vi "Cleanup.vi"(8 "error in (no error)":errorcluster, 11 "SQLite in":refnum<class "SQLite.lvclass">) -> (0 "error out":errorcluster)   [LabVIEW 2020, in "Summer of LabVIEW.lvlib" / "SQLite.lvclass"]
uses:
  SQLite.lvclass
  SQLite.lvclass/SQLite.ctl
  <vilib>/drjdpowell/SQLite Library/SQL Connection/Connection.lvclass
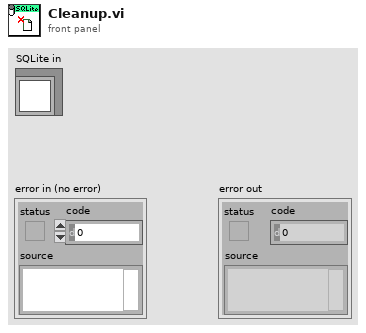
[diagram p1: front panel]
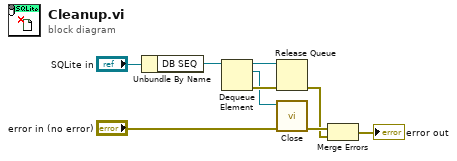
[diagram p0: block diagram]
diagram:
  n1 = Unbundle By Name("SQLite in") -> ("DB SEQ"=w8:refnum<queue>)
  n2 = Dequeue Element(queue=w8) -> (queue out=w7:refnum<queue>, element=w4:refnum<class "Connection.lvclass">, error out=w6:errorcluster)  [unwired: 2 in, 1 out]
  n3 = Release Queue(queue=w7, error in (no error)=w6) -> (error out=w2:errorcluster)  [unwired: 1 in, 2 out]
  n4 = call-dynamic "Close.vi"("error in (no error)"="error in (no error)", "SQLite Connection in"=w4) -> ("error out"=w3:errorcluster)  [unwired: 9 in]
  n5 = Merge Errors(w3, w2) -> (→"error out":errorcluster)
